vi "Calculate Rate from Num Channels and Max Rate.vi"(8 "error in (no error)":errorcluster, 10 "Channel Data Rate S/s":dbl, 11 "Number of Channels":i32) -> (0 "error out":errorcluster, 3 "Rate":dbl)   [LabVIEW 2015]
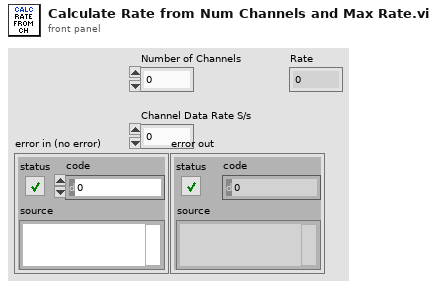
[diagram p1: front panel]
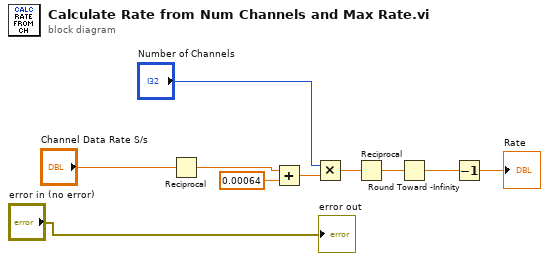
[diagram p0: block diagram]
diagram:
  n1 = Reciprocal(x="Channel Data Rate S/s") -> (1/x=w3:dbl)
  n2 = Add(x=w3, y=0.00064) -> (x+y=w4:dbl)
  n3 = Multiply(x="Number of Channels", y=w4) -> (x*y=w9:dbl)
  n4 = Reciprocal(x=w9) -> (1/x=w6:dbl)
  n5 = Round Toward -Infinity(1:w6) -> (0:w7:dbl)
  n6 = Decrement(x=w7) -> (x-1=→"Rate":dbl)
  "error out" <- "error in (no error)"
